vi "merlinEngine.vi"() -> ()   [LabVIEW 2018]
uses:
  classes/Tushars Events Toolkit/Software/Modules/EventClient_ObjectReference.ctl
  classes/Variable Manager/VariableManager_Bool.vi
  Strict Type Controls/Settings Operation.ctl
  <vilib>/Instr/_visa.llb/VISA Configure Serial Port (Instr).vi
  classes/Variable Manager/VariableManager_Double.vi
panel:
  out "Value":dbl
  out "Quit":bool
  out "error out":errorcluster
  in  "error in (no error)":errorcluster
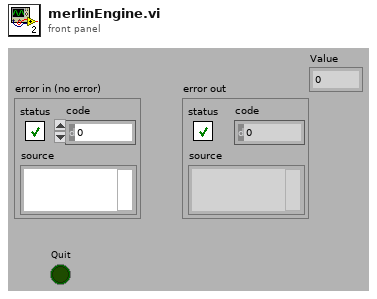
[diagram p1: front panel]
types:
  T1 = enum16{"Int Chop Off", "Int Chop On", "Ext Chop Off", "Ext Chop On"}
  T2 = cluster{"Merlin.Port":refnum<visa-resource-name>}
  T3 = typedef "EventClient_ObjectReference.ctl" = refnum<k1>
  T4 = typedef "Settings Operation.ctl" = enum8{"Get Value", "Set Value", "Read File", "Write File", "Write Stored Value"}
  T5 = cluster{"#Stages":enum16{"None", "1 Pole", "2 Pole"}, "Phase":enum16{"1 Phase", "2 Phase"}, "SyncMode":enum16{"Int Chop Off", "Int Chop On", "Ext Chop Off", "Ext Chop On"}, "Time Const":enum16{".003s", ".010s", ".030s", ".100s", ".300s", "1.00s", "3.00s", "10.0s", "30.0s", "100s"}, "Frequency":u32}
  T6 = typedef "Settings.ctl" = cluster{"Mono Cr":cluster{"Port":refnum<visa-resource-name>, "baud rate":u32, "data bits":u16, "parity":enum16{"None", "Odd", "Even", "Mark", "Space"}, "stop bits":u16, "flow control":u16, "timeout":u32}, "Merlin":cluster{"Port":refnum<visa-resource-name>, "baud rate":u32, "data bits":u16, "parity":enum16{"None", "Odd", "Even", "Mark", "Space"}, "stop bits":u16, "flow control":u16, "timeout":u32}}
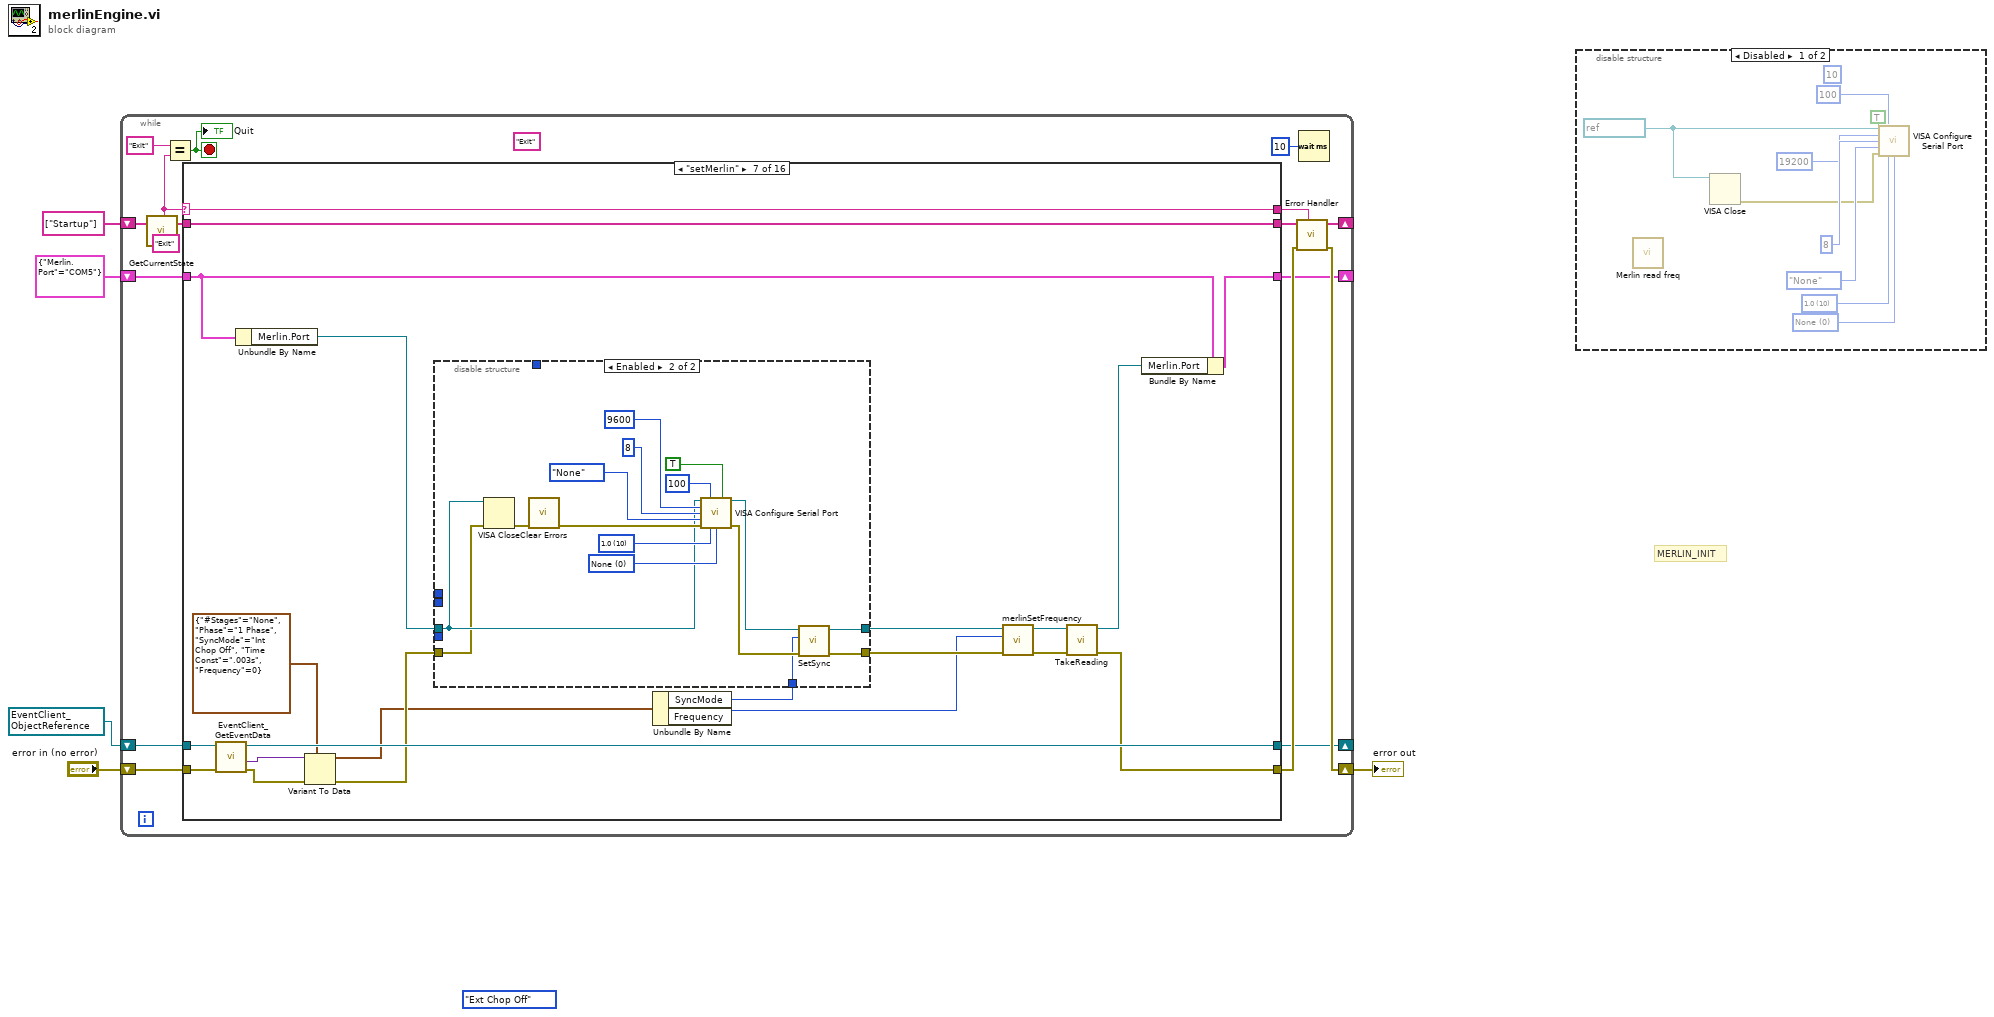
[diagram p0: block diagram]
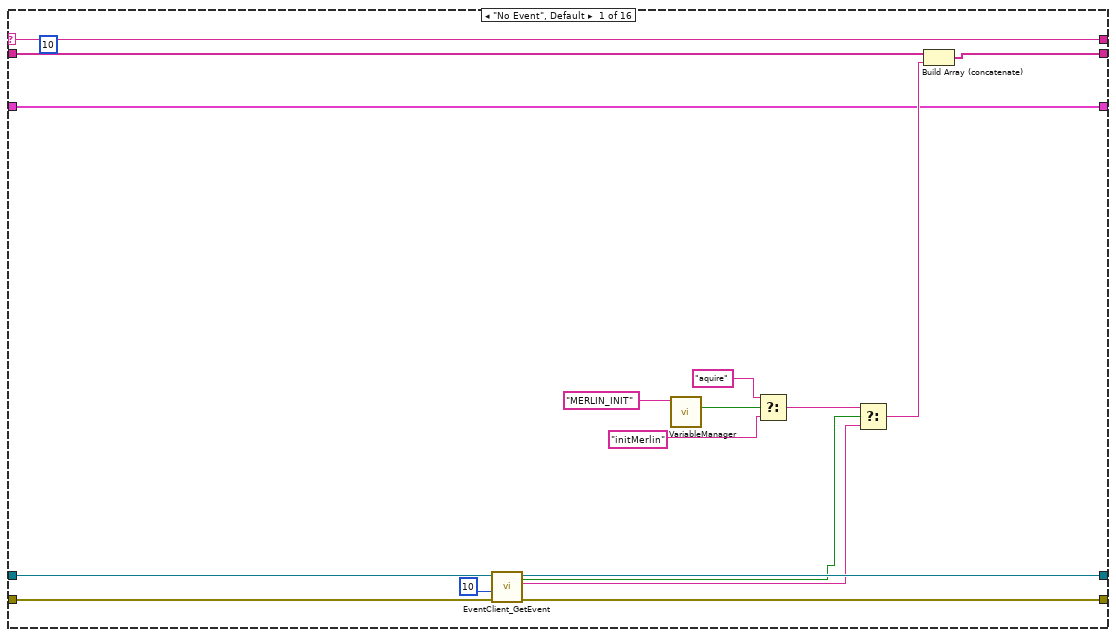
[diagram p3: hidden frame]
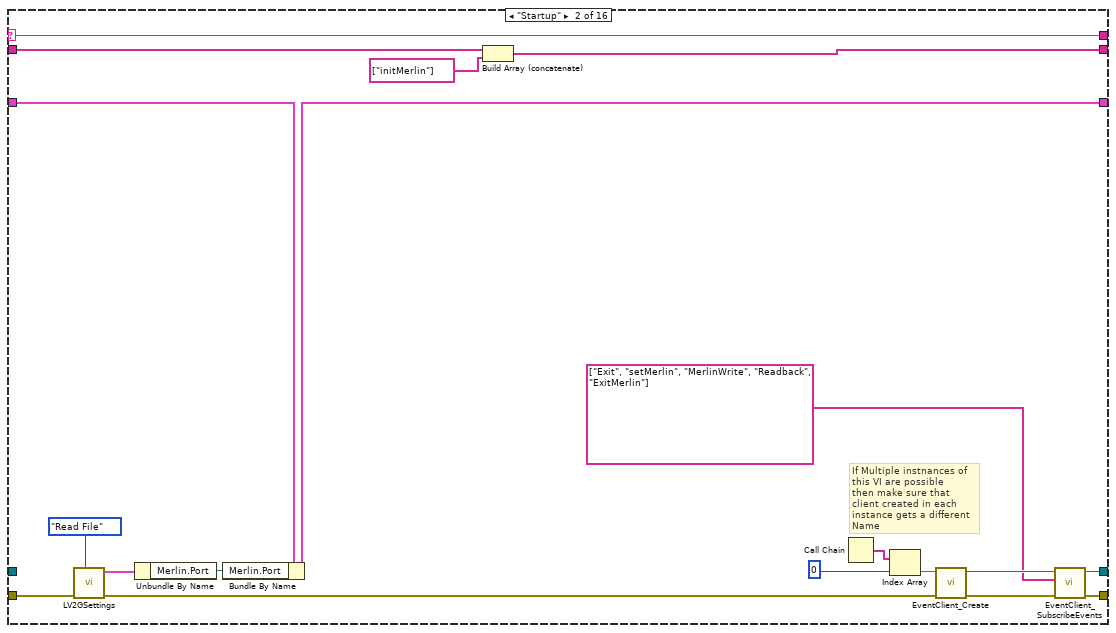
[diagram p4: hidden frame]
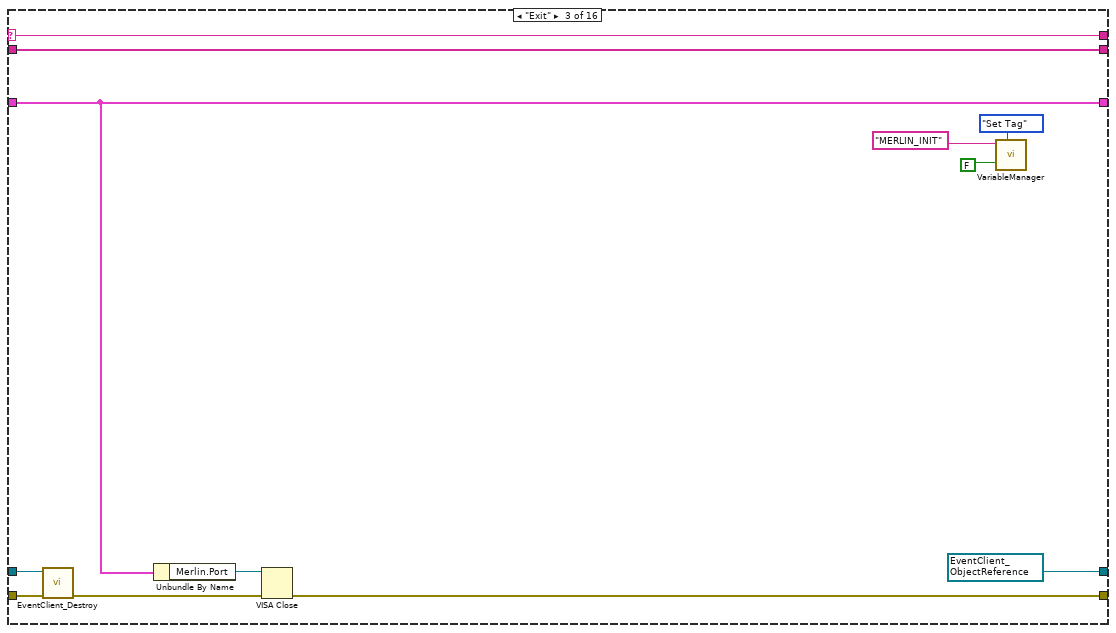
[diagram p5: hidden frame]
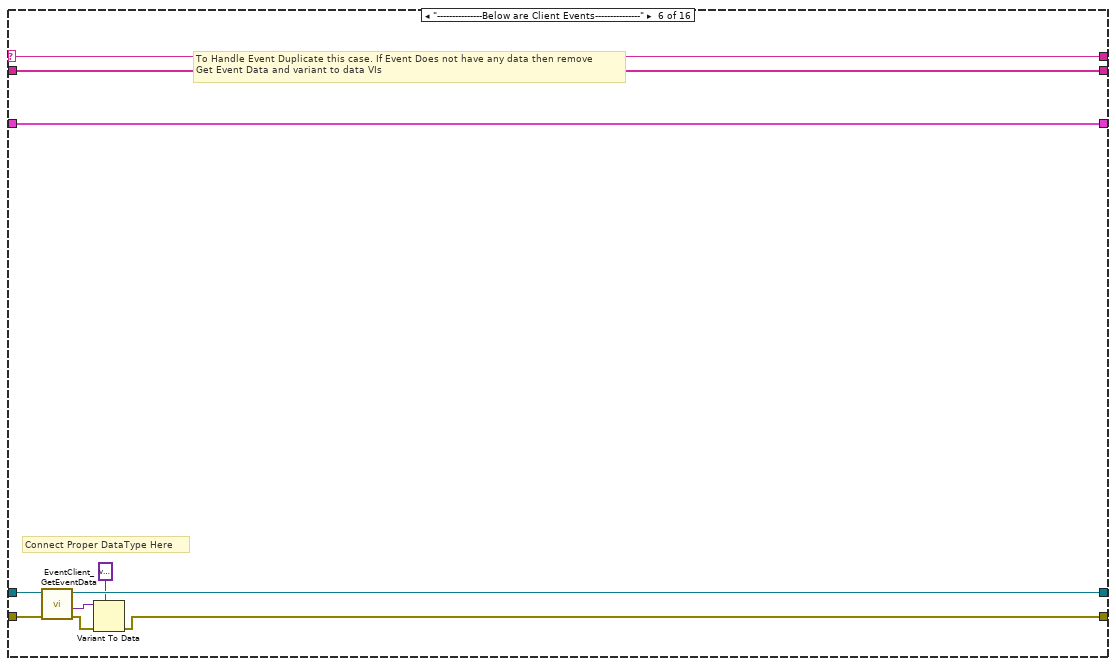
[diagram p8: hidden frame]
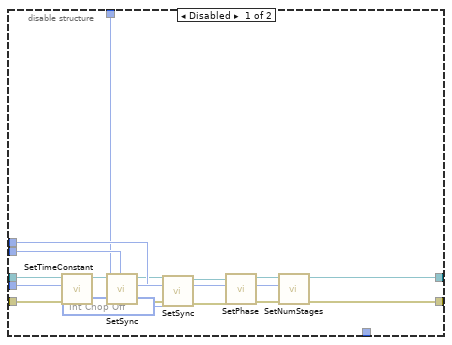
[diagram p9: hidden frame]
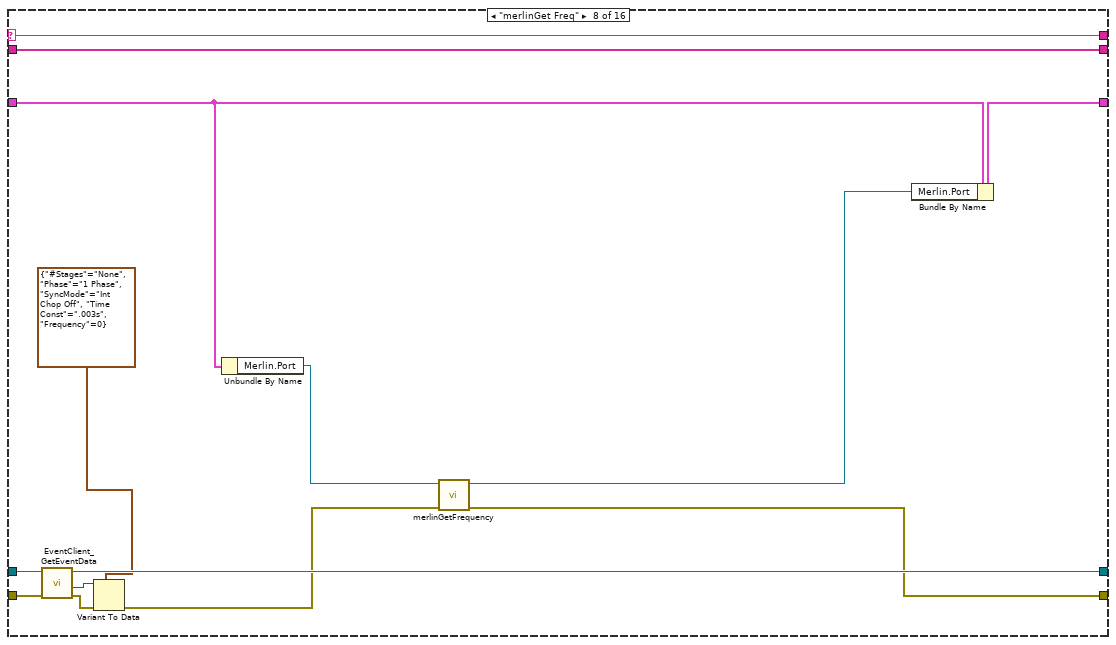
[diagram p10: hidden frame]
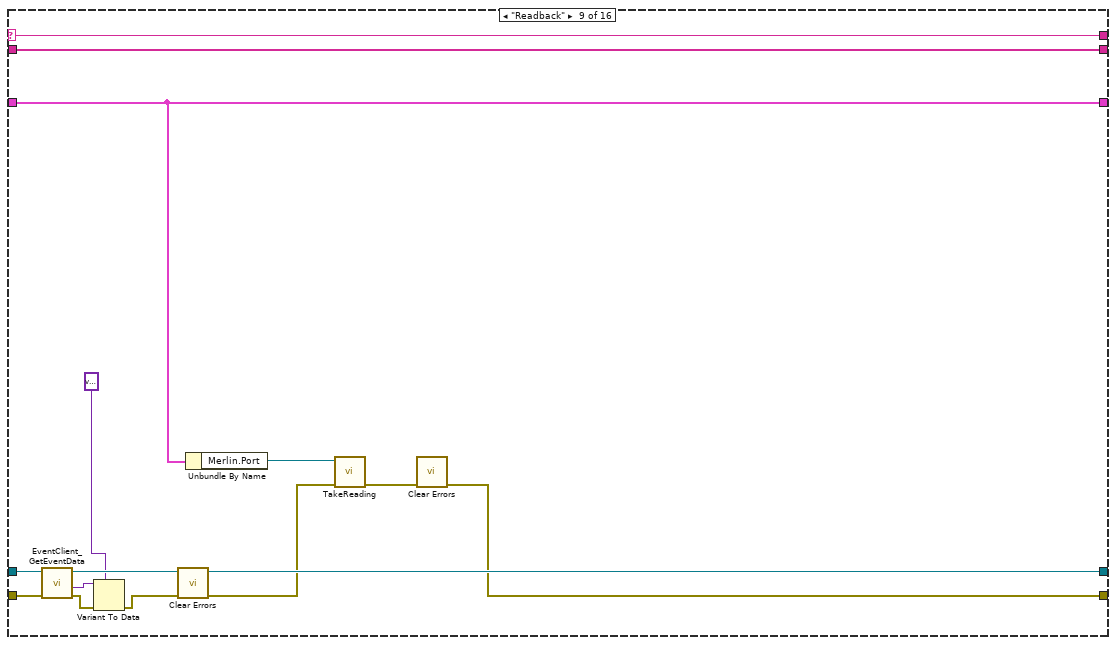
[diagram p11: hidden frame]
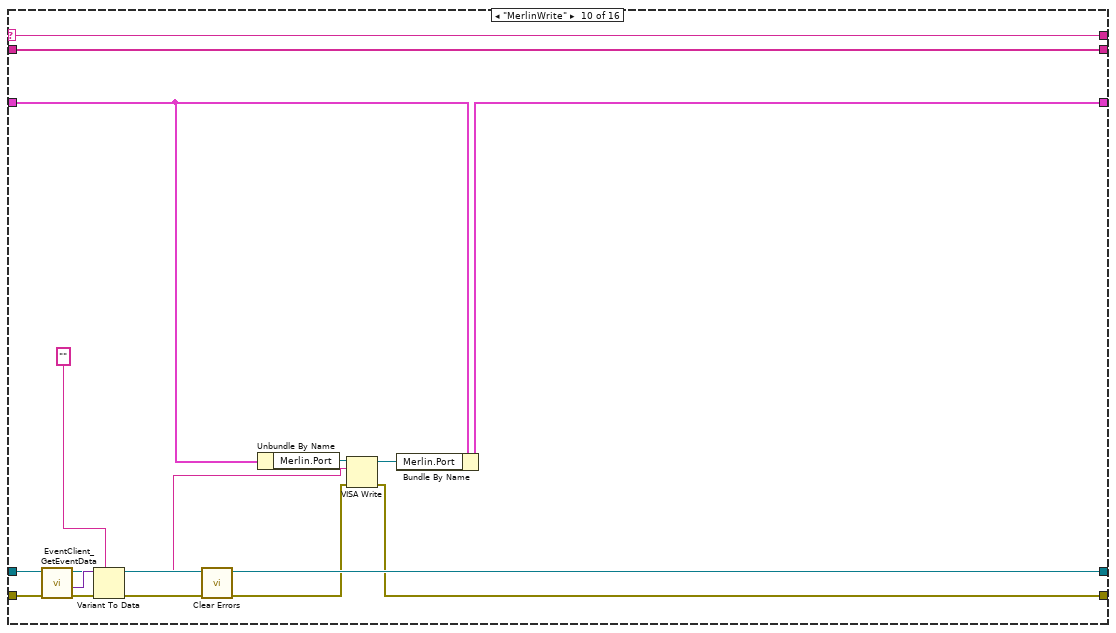
[diagram p12: hidden frame]
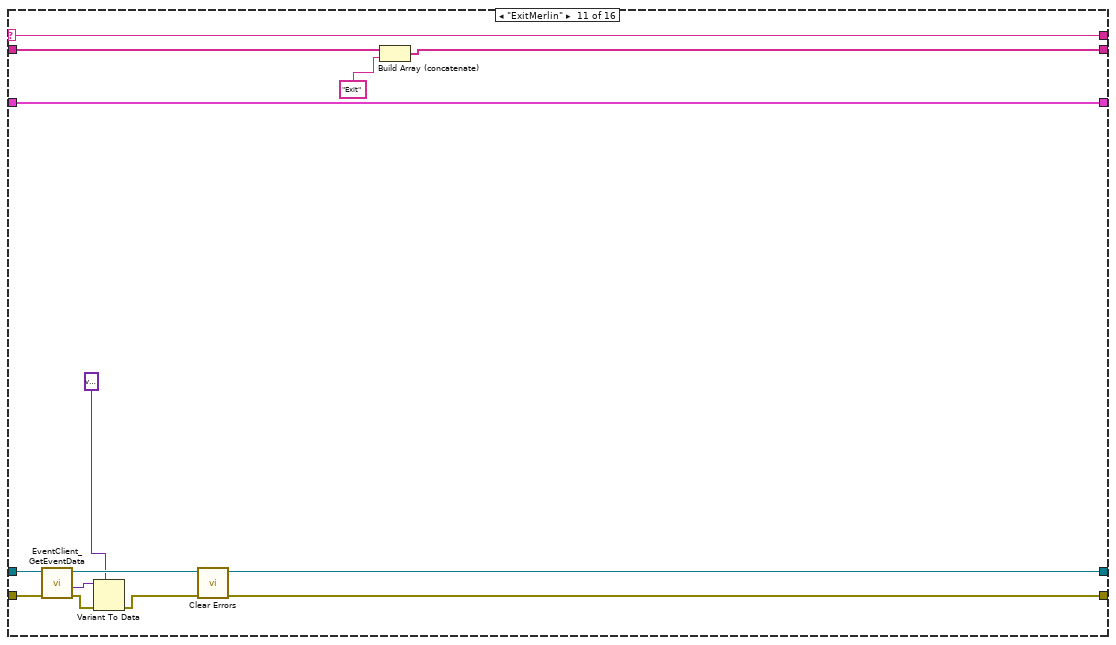
[diagram p13: hidden frame]
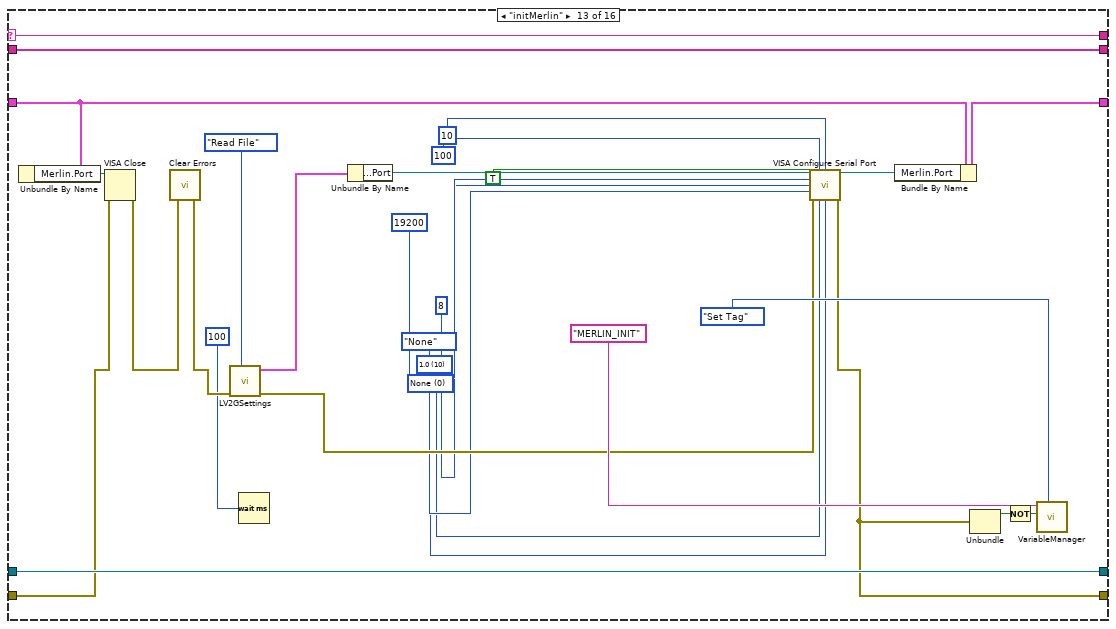
[diagram p15: hidden frame]
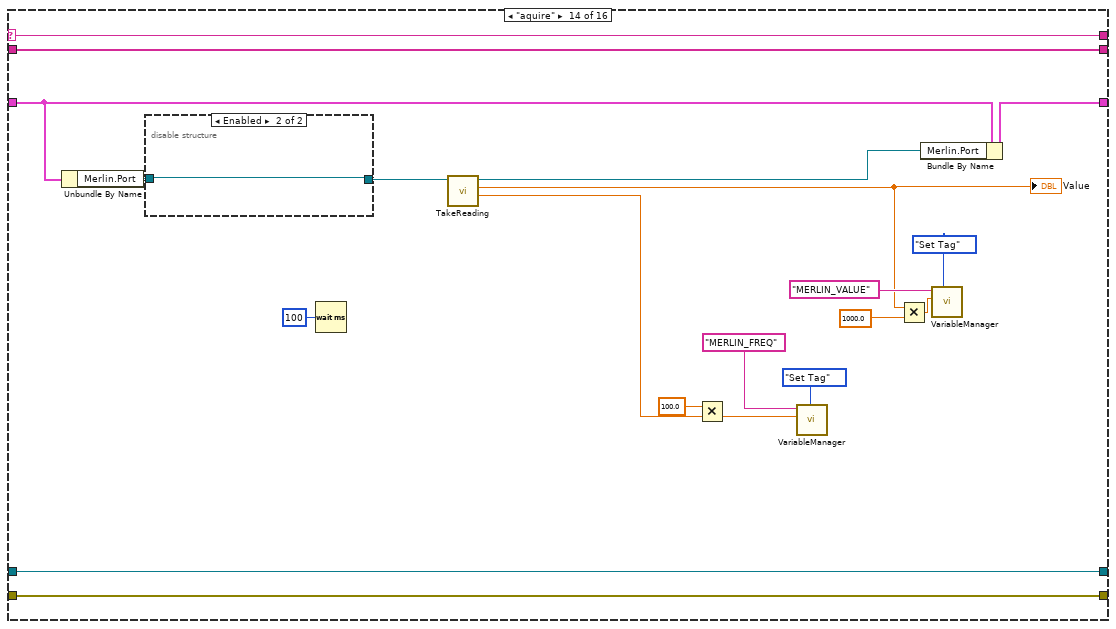
[diagram p16: hidden frame]
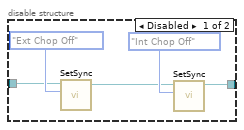
[diagram p17: hidden frame]
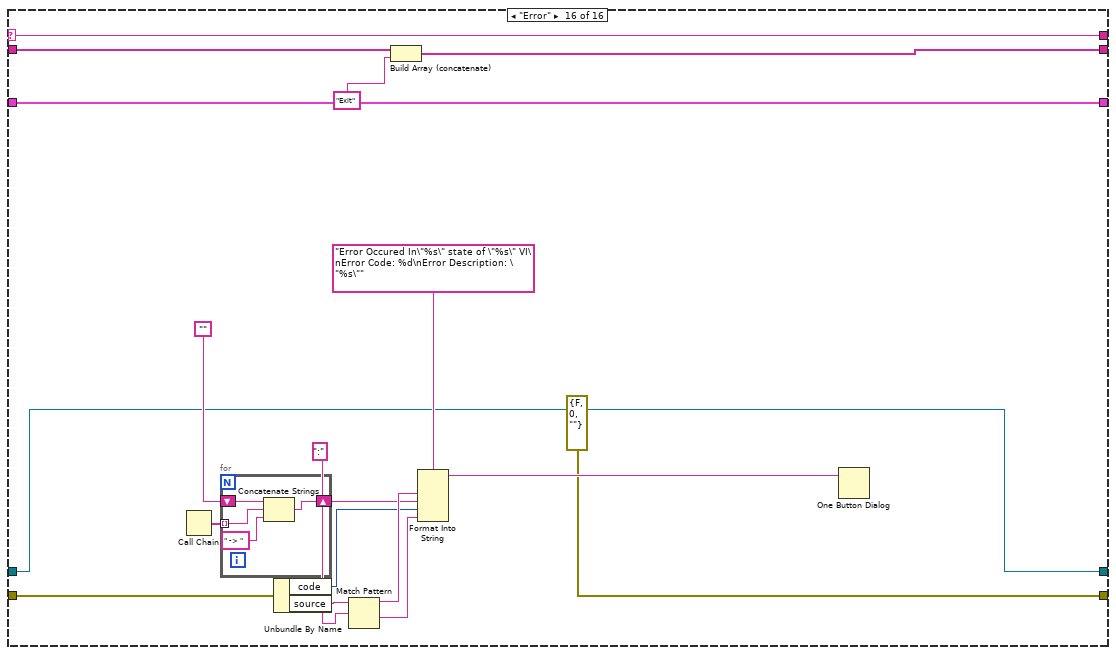
[diagram p19: hidden frame]
diagram:
  (unwired) T1."Ext Chop Off" ("SyncMode")
  w2 = T3 refnum items=["EventClient"] ("reference")
  # "MERLIN_INIT"
  n1 = while {
    shift-right: [w17] -> _
    shift-left: string[] ["Startup"] ("State Array Out") -> [w21]
    shift-right: [w13] -> w3
    shift-left: "error in (no error)" -> [w14]
    shift-right: [w10] -> _
    shift-left: w2 -> [w9]
    shift-right: [w8] -> _
    shift-left: T2 {"Merlin.Port"="COM5"} -> [w7]
    stop <- w18 stop-if-true
    (unwired) "Exit" ("x")
    (unwired) "Exit" ("x")
    n2 = call "GetCurrentState.vi"("State Array In"=w21) -> ("Current State"=w11:string, "State Array Out"=w20:string[])  [unwired: 17 in]
    n3 = Equal?(x="Exit", y=w11) -> (x = y?=w18:bool)
    "Quit" <- w18
    n4 = case shown="\"setMerlin\"" w11 {
      selector: w11 -> [w38 w57 w69 w73 w78 w88 w109 w156 w170 w186 w199 w204 w232 w252 w264 w282]
      tunnel: w20 -> [w26 w56 w68 w74 w79 w89 w110 w157 w171 w187 w200 w205 w233 w253 w263 w269]
      tunnel: [w25 w55 w68 w74 w79 w89 w110 w157 w171 w187 w190 w205 w233 w253 w263 w266] -> w16
      tunnel: [w35 w49 w58 w72 w77 w84 w91 w146 w158 w173 w188 w203 w218 w251 w262 errorcluster {"status"=FALSE, "code"=0, "source"=""} ("error in (no error)")] -> w12
      tunnel: [w38 w57 w69 w73 w78 w88 w109 w156 w170 w186 w199 w204 w232 w252 w264 w282] -> w15
      tunnel: w14 -> [w36 w45 w66 w72 w77 w86 w107 w154 w168 w184 w197 w203 w215 w251 w262 w270]
      tunnel: [w34 w47 w65 w71 w76 w82 w104 w151 w164 w180 w193 w202 w231 w250 w261 w268] -> w10
      tunnel: w9 -> [w37 _ w67 w71 w76 w87 w108 w155 w169 w185 w198 w202 w231 w250 w261 w268]
      tunnel: [w22 w41 w61 w70 w75 w80 w101 w149 w160 w176 w191 w201 w219 w244 w260 w267] -> w8
      tunnel: w7 -> [w22 w42 w61 w70 w75 w80 w102 w150 w160 w177 w191 w201 w220 w245 w260 w267]
      frame "No Event", Default {
        (unwired) 10
        n5 = call "EventClient_GetEvent.vi"("error in (no error)"=w36, "timeout in ms (-1)"=10, "reference"=w37) -> ("error out"=w35:errorcluster, "Name"=w23:string, "reference out"=w34:T3, "timed out?"=w27:bool)  [unwired: 4 in, 1 out]
        n6 = call-poly "VariableManager.vi"("Tag"="MERLIN_INIT") -> ("Value out"=w31:bool)  [unwired: 7 in, 3 out]
        n7 = Select(t="aquire" ("Tag"), s=w31, f="initMerlin" ("Tag")) -> (s? t:f=w28:string)
        n8 = Select(t=w28, s=w27, f=w23) -> (s? t:f=w24:string)
        n9 = Build Array (concatenate)(w26, w24) -> (w25:string[])
      }
      frame "Startup" {
        # "If Multiple instnances of this VI are possible \nthen make sure that client created in each instance gets a different Name"
        n10 = call "LV2GSettings.vi"("Operation"=Settings_Operation."Read File", "error in (no error)"=w45) -> ("error out"=w44:errorcluster, "Settings out"=w40:T6)  [unwired: 8 in]
        n11 = Unbundle By Name(w40) -> ("Merlin.Port"=w39:refnum<visa-resource-name>)
        n12 = Bundle By Name(cluster=w42, "Merlin.Port"=w39) -> (w41:T2)
        n13 = Build Array (concatenate)(w56, string[] ["initMerlin"] ("State Array Out")) -> (w55:string[])
        n14 = Call Chain() -> (call chain=w53:string[])
        n15 = Index Array(array=w53, index=0) -> (element=w51:string)
        n16 = call "EventClient_Create.vi"("error in (no error)"=w44, "Instance Name"=w51) -> ("error out"=w50:errorcluster, "reference"=w48:T3)  [unwired: 8 in]
        n17 = call "EventClient_SubscribeEvents.vi"("error in (no error)"=w50, "Events"=string[] ["Exit", "setMerlin", "MerlinWrite", "Readback", "ExitMerlin"], "reference"=w48) -> ("error out"=w49:errorcluster, "reference out"=w47:T3)  [unwired: 7 in]
      }
      frame "Exit" {
        w65 = T3 refnum items=["EventClient"] ("reference out")
        n18 = call "EventClient_Destroy.vi"("error in (no error)"=w66, "reference"=w67) -> ("error out"=w59:errorcluster)  [unwired: 9 in]
        n19 = Unbundle By Name(w61) -> ("Merlin.Port"=w60:refnum<visa-resource-name>)
        n20 = VISA Close(VISA resource name=w60, error in (no error)=w59) -> (error out=w58:errorcluster)
        n21 = call-poly "VariableManager.vi"("Operation"=enum16{"Get Tag", "Set Tag"}."Set Tag", "Value"=FALSE, "Tag"="MERLIN_INIT") -> ()  [unwired: 5 in, 4 out]
      }
      frame "---------------Below are UI Events---------------" {
        # "This State will never Execute\nIt is added just for improving code readability please do not remove this case"
      }
      frame "---------------Below are Menu Events---------------" {
        # "This State will never Execute\nIt is added just for improving code readability please do not remove this case"
      }
      frame "---------------Below are Client Events---------------" {
        # "To Handle Event Duplicate this case. If Event Does not have any data then remove\nGet Event Data and variant to data VIs"
        # "Connect Proper DataType Here"
        n22 = call "EventClient_GetEventData.vi"("error in (no error)"=w86, "reference"=w87) -> ("error out"=w85:errorcluster, "Data"=w83:variant, "reference out"=w82:T3)  [unwired: 7 in]
        n23 = Variant To Data(error in=w85, type=variant, Variant=w83) -> (error out=w84:errorcluster)  [unwired: 1 out]
      }
      frame "setMerlin" {
        n24 = call "EventClient_GetEventData.vi"("error in (no error)"=w107, "reference"=w108) -> ("error out"=w106:errorcluster, "Data"=w105:variant, "reference out"=w104:T3)  [unwired: 7 in]
        n25 = Unbundle By Name(w102) -> ("Merlin.Port"=w103:refnum<visa-resource-name>)
        n26 = Variant To Data(error in=w106, type=T5 {"#Stages"=enum."None", "Phase"=enum."1 Phase", "SyncMode"=enum."Int Chop Off", "Time Const"=enum.".003s", "Frequency"=0}, Variant=w105) -> (data=w96:T5, error out=w100:errorcluster)
        n27 = Unbundle By Name(w96) -> ("SyncMode"=w90:T1, "Frequency"=w95:u32)
        n28 = disable-structure shown="Enabled" {
          disable-tunnel: _ -> [w125 _]
          disable-tunnel: w103 -> [w124 w134]
          disable-tunnel: _ -> [w121 _]
          disable-tunnel: _ -> [w120 _]
          disable-tunnel: w100 -> [w119 w128]
          disable-tunnel: [w118 w132] -> w98
          disable-tunnel: [w117 w131] -> w97
          disable-tunnel: _ -> [w116 _]
          disable-tunnel: w90 -> [_ w129]
          frame Disabled {
            n29 = call "SetTimeConstant.vi"("error in"=w119, "Time Const"=w125, "Port"=w124) -> ("error out"=w127:errorcluster, "Port out"=w123:refnum<visa-resource-name>)  [unwired: 7 in]
            n30 = call "SetSync.vi"("error in"=w127, "SyncMode"=w116, "Port"=w123) -> ("error out"=w113:errorcluster, "Port out"=w115:refnum<visa-resource-name>)  [unwired: 7 in]
            n31 = call "SetSync.vi"("error in"=w113, "SyncMode"=T1."Int Chop Off", "Port"=w115) -> ("error out"=w112:errorcluster, "Port out"=w114:refnum<visa-resource-name>)  [unwired: 7 in]
            n32 = call "SetPhase.vi"("error in"=w112, "Phase"=w121, "Port"=w114) -> ("error out"=w126:errorcluster, "Port out"=w122:refnum<visa-resource-name>)  [unwired: 7 in]
            n33 = call "SetNumStages.vi"("error in"=w126, "#Stages"=w120, "Port"=w122) -> ("error out"=w118:errorcluster, "Port out"=w117:refnum<visa-resource-name>)  [unwired: 7 in]
          }
          frame Enabled {
            w135 = u16 0 items=["None", "XON/XOFF", "RTS/CTS", "XON/XOFF & RTS/CTS", "DTR/DSR", "XON/XOFF & DTR/DSR"] ("flow control (0:none)")
            w136 = u16 10 items=["1.0"=10, "1.5"=15, "2.0"=20] ("stop bits (10: 1 bit)")
            n34 = VISA Close(VISA resource name=w134, error in (no error)=w128) -> (error out=w142:errorcluster)
            n35 = call <vilib>:"Clear Errors.vi"("error in (no error)"=w142) -> ("error out"=w143:errorcluster)  [unwired: 5 in, 1 out]
            n36 = call-poly "VISA Configure Serial Port"("VISA resource name"=w134, "timeout (10sec)"=u32 100, "Enable Termination\nChar (T)"=TRUE ("Enable Termination\nChar (T)"), "baud rate (9600)"=u32 9600, "data bits (8)"=u16 8, "parity (0:none)"=enum16{"None", "Odd", "Even", "Mark", "Space"}."None", "error in (no error)"=w143, "stop bits (10: 1 bit)"=w136, "flow control (0:none)"=w135) -> ("VISA resource name out"=w130:refnum<visa-resource-name>, "error out"=w133:errorcluster)  [unwired: 5 in]
            n37 = call "SetSync.vi"("error in"=w133, "SyncMode"=w129, "Port"=w130) -> ("error out"=w132:errorcluster, "Port out"=w131:refnum<visa-resource-name>)  [unwired: 7 in]
          }
        }
        n38 = call "merlinSetFrequency.vi"("error in"=w98, "Freq"=w95, "Port"=w97) -> ("error out"=w92:errorcluster, "Port out"=w94:refnum<visa-resource-name>)  [unwired: 7 in]
        n39 = call "TakeReading.vi"("error in"=w92, "Port"=w94) -> ("error out"=w91:errorcluster, "Port out"=w93:refnum<visa-resource-name>)  [unwired: 6 in, 2 out]
        n40 = Bundle By Name(cluster=w102, "Merlin.Port"=w93) -> (w101:T2)
      }
      frame "merlinGet Freq" {
        n41 = call "EventClient_GetEventData.vi"("error in (no error)"=w154, "reference"=w155) -> ("error out"=w153:errorcluster, "Data"=w152:variant, "reference out"=w151:T3)  [unwired: 7 in]
        n42 = Variant To Data(error in=w153, type=T5 {"#Stages"=enum."None", "Phase"=enum."1 Phase", "SyncMode"=enum."Int Chop Off", "Time Const"=enum.".003s", "Frequency"=0}, Variant=w152) -> (error out=w147:errorcluster)  [unwired: 1 out]
        n43 = Unbundle By Name(w150) -> ("Merlin.Port"=w145:refnum<visa-resource-name>)
        n44 = call "merlinGetFrequency.vi"("error in"=w147, "Port"=w145) -> ("error out"=w146:errorcluster, "Port out"=w144:refnum<visa-resource-name>)  [unwired: 7 in, 1 out]
        n45 = Bundle By Name(cluster=w150, "Merlin.Port"=w144) -> (w149:T2)
      }
      frame "Readback" {
        n46 = call "EventClient_GetEventData.vi"("error in (no error)"=w168, "reference"=w169) -> ("error out"=w167:errorcluster, "Data"=w165:variant, "reference out"=w164:T3)  [unwired: 7 in]
        n47 = Variant To Data(error in=w167, type=variant, Variant=w165) -> (error out=w166:errorcluster)  [unwired: 1 out]
        n48 = call <vilib>:"Clear Errors.vi"("error in (no error)"=w166) -> ("error out"=w159:errorcluster)  [unwired: 5 in, 1 out]
        n49 = Unbundle By Name(w160) -> ("Merlin.Port"=w162:refnum<visa-resource-name>)
        n50 = call "TakeReading.vi"("error in"=w159, "Port"=w162) -> ("error out"=w161:errorcluster)  [unwired: 6 in, 3 out]
        n51 = call <vilib>:"Clear Errors.vi"("error in (no error)"=w161) -> ("error out"=w158:errorcluster)  [unwired: 5 in, 1 out]
      }
      frame "MerlinWrite" {
        n52 = call "EventClient_GetEventData.vi"("error in (no error)"=w184, "reference"=w185) -> ("error out"=w183:errorcluster, "Data"=w181:variant, "reference out"=w180:T3)  [unwired: 7 in]
        n53 = Variant To Data(error in=w183, type="", Variant=w181) -> (data=w172:string, error out=w182:errorcluster)
        n54 = call <vilib>:"Clear Errors.vi"("error in (no error)"=w182) -> ("error out"=w174:errorcluster)  [unwired: 5 in, 1 out]
        n55 = Unbundle By Name(w177) -> ("Merlin.Port"=w179:refnum<visa-resource-name>)
        n56 = VISA Write(VISA resource name=w179, write buffer=w172, error in (no error)=w174) -> (VISA resource name out=w175:refnum<visa-resource-name>, error out=w173:errorcluster)  [unwired: 1 out]
        n57 = Bundle By Name(cluster=w177, "Merlin.Port"=w175) -> (w176:T2)
      }
      frame "ExitMerlin" {
        n58 = call "EventClient_GetEventData.vi"("error in (no error)"=w197, "reference"=w198) -> ("error out"=w196:errorcluster, "Data"=w194:variant, "reference out"=w193:T3)  [unwired: 7 in]
        n59 = Variant To Data(error in=w196, type=variant, Variant=w194) -> (error out=w195:errorcluster)  [unwired: 1 out]
        n60 = call <vilib>:"Clear Errors.vi"("error in (no error)"=w195) -> ("error out"=w188:errorcluster)  [unwired: 5 in, 1 out]
        n61 = Build Array (concatenate)(w200, "Exit" ("x")) -> (w190:string[])
      }
      frame "---------------Below are Subroutine states---------------" {
      }
      frame "initMerlin" {
        w207 = u16 0 items=["None", "XON/XOFF", "RTS/CTS", "XON/XOFF & RTS/CTS", "DTR/DSR", "XON/XOFF & DTR/DSR"] ("flow control (0:none)")
        w208 = u16 10 items=["1.0"=10, "1.5"=15, "2.0"=20] ("stop bits (10: 1 bit)")
        n62 = Unbundle By Name(w220) -> ("Merlin.Port"=w227:refnum<visa-resource-name>)
        n63 = VISA Close(VISA resource name=w227, error in (no error)=w215) -> (error out=w229:errorcluster)
        n64 = call <vilib>:"Clear Errors.vi"("error in (no error)"=w229) -> ("error out"=w228:errorcluster)  [unwired: 5 in, 1 out]
        n65 = call "LV2GSettings.vi"("Operation"=Settings_Operation."Read File", "error in (no error)"=w228) -> ("error out"=w216:errorcluster, "Settings out"=w230:T6)  [unwired: 8 in]
        n66 = Wait (ms)(milliseconds to wait=u32 100) -> ()  [unwired: 1 out]
        n67 = Unbundle By Name(w230) -> ("Merlin.Port"=w206:refnum<visa-resource-name>)
        n68 = call-poly "VISA Configure Serial Port"("VISA resource name"=w206, "timeout (10sec)"=u32 100, "termination char\n(0xA = '\\n' = LF)"=u8 10 ("termination char\n(0xA = '\\n' = LF)"), "Enable Termination\nChar (T)"=TRUE ("Enable Termination\nChar (T)"), "baud rate (9600)"=u32 19200, "data bits (8)"=u16 8, "parity (0:none)"=enum16{"None", "Odd", "Even", "Mark", "Space"}."None", "error in (no error)"=w216, "stop bits (10: 1 bit)"=w208, "flow control (0:none)"=w207) -> ("VISA resource name out"=w226:refnum<visa-resource-name>, "error out"=w218:errorcluster)  [unwired: 4 in]
        n69 = Bundle By Name(cluster=w220, "Merlin.Port"=w226) -> (w219:T2)
        n70 = Unbundle(w218) -> ("status"=w224:bool)  [unwired: 2 out]
        n71 = Not(x=w224) -> (.not. x?=w225:bool)
        n72 = call-poly "VariableManager.vi"("Operation"=enum16{"Get Tag", "Set Tag"}."Set Tag", "Value"=w225, "Tag"="MERLIN_INIT") -> ()  [unwired: 5 in, 4 out]
      }
      frame "aquire" {
        n73 = Unbundle By Name(w245) -> ("Merlin.Port"=w238:refnum<visa-resource-name>)
        n74 = disable-structure shown="Enabled" {
          disable-tunnel: w238 -> [w257 w259]
          disable-tunnel: [w254 w259] -> w237
          frame Disabled {
            n75 = call "SetSync.vi"("SyncMode"=T1."Ext Chop Off", "Port"=w257) -> ("Port out"=w255:refnum<visa-resource-name>)  [unwired: 8 in, 1 out]
            n76 = call "SetSync.vi"("SyncMode"=T1."Int Chop Off", "Port"=w255) -> ("Port out"=w254:refnum<visa-resource-name>)  [unwired: 8 in, 1 out]
          }
          frame Enabled {
          }
        }
        n77 = Wait (ms)(milliseconds to wait=u32 100) -> ()  [unwired: 1 out]
        n78 = call "TakeReading.vi"("Port"=w237) -> ("Frequency"=w239:dbl, "Voltage(mV)"=w246:dbl, "Port out"=w249:refnum<visa-resource-name>)  [unwired: 7 in, 1 out]
        "Value" <- w246
        n79 = Multiply(x=100.0, y=w239) -> (x*y=w236:dbl)
        n80 = call-poly "VariableManager.vi"("Operation"=enum16{"Get Tag", "Set Tag"}."Set Tag", "Value"=w236, "Tag"="MERLIN_FREQ") -> ()  [unwired: 4 in, 5 out]
        n81 = Multiply(x=w246, y=1000.0 ("x")) -> (x*y=w243:dbl)
        n82 = Bundle By Name(cluster=w245, "Merlin.Port"=w249) -> (w244:T2)
        n83 = call-poly "VariableManager.vi"("Operation"=enum16{"Get Tag", "Set Tag"}."Set Tag", "Value"=w243, "Tag"="MERLIN_VALUE") -> ()  [unwired: 4 in, 5 out]
      }
      frame "---------------Below are Error Handling VIs---------------" {
      }
      frame "Error" {
        n84 = Call Chain() -> (call chain=w277:string[])
        n85 = for {
          tunnel: w277 -> [w285] mode=indexing
          shift-right: [w283] -> w274
          shift-left: "" -> [w286]
          n86 = Concatenate Strings(w286, w285, " -> ") -> (w283:string)
        }
        n87 = Unbundle By Name(w270) -> ("code"=w272:i32, "source"=w271:string)
        n88 = Match Pattern(string=w271, regular expression=":") -> (before substring=w275:string, after substring=w279:string)  [unwired: 1 in, 2 out]
        n89 = Build Array (concatenate)(w269, "Exit" ("x")) -> (w266:string[])
        n90 = Format Into String(format string="Error Occured In\"%s\" state of \"%s\" VI\nError Code: %d\nError Description: \"%s\"", w275, w274, w272, w279) -> (resulting string=w278:string)  [unwired: 2 in, 1 out]
        n91 = One Button Dialog(message=w278) -> ()  [unwired: 1 in, 1 out]
      }
    }
    n92 = call "Error Handler.vi"("Current State"=w15, "error in (no error)"=w12, "Msg Queue In"=w16) -> ("error out"=w13:errorcluster, "Msg Queue Out"=w17:string[])  [unwired: 7 in]
    n93 = Wait (ms)(milliseconds to wait=u32 10) -> ()  [unwired: 1 out]
  }
  "error out" <- w3
  n94 = disable-structure shown="Disabled" {
    frame Disabled {
      w288 = refnum<visa-resource-name> "COM4" ("VISA resource name")
      w295 = u16 0 items=["None", "XON/XOFF", "RTS/CTS", "XON/XOFF & RTS/CTS", "DTR/DSR", "XON/XOFF & DTR/DSR"] ("flow control (0:none)")
      w294 = u16 10 items=["1.0"=10, "1.5"=15, "2.0"=20] ("stop bits (10: 1 bit)")
      (unwired) u8 10 ("termination char\n(0xA = '\\n' = LF)")
      n95 = call "Merlin read freq.vi"() -> ()  [unwired: 11 in, 1 out]
      n96 = VISA Close(VISA resource name=w288) -> (error out=w287:errorcluster)  [unwired: 1 in]
      n97 = call-poly "VISA Configure Serial Port"("VISA resource name"=w288, "timeout (10sec)"=u32 100, "Enable Termination\nChar (T)"=TRUE ("Enable Termination\nChar (T)"), "baud rate (9600)"=u32 19200, "data bits (8)"=u16 8, "parity (0:none)"=enum16{"None", "Odd", "Even", "Mark", "Space"}."None", "error in (no error)"=w287, "stop bits (10: 1 bit)"=w294, "flow control (0:none)"=w295) -> ()  [unwired: 5 in, 2 out]
    }
    frame Enabled {
    }
  }
